vi "3d surface.vi"() -> ()   [LabVIEW 2012]
uses:
  <vilib>/Native 3D Graph/xcontrol/3DPC_SurfacePlot.xctl
  <vilib>/imath/engines/lvmath2/RunTimeEngine/ErrorHandling/NIMS_Finalize Error.vi
  <vilib>/imath/engines/lvmath2/RunTimeEngine/NodeEndStatement/NIMS_NodeEndStatement_Output.vi
  <instcachedir>/0/NIMS_NodeEndStatement_Output_53EC0D466D134D7ABD903AC30B43404B.lvgen/NIMS_NodeEndStatement_Output_53EC0D466D134D7ABD903AC30B43404B_002.vi
  <vilib>/imath/engines/lvmath2/RunTimeEngine/BuiltInFunctions/peakfcn2d/NIMS_peakfcn2d(I32S).vi
  <vilib>/imath/engines/lvmath2/RunTimeEngine/ErrorHandling/NIMS_Error From Error Code.vi
  <vilib>/imath/engines/lvmath2/RunTimeEngine/BuiltInFunctions/surface/NIMS_surface(RM, RM).vi
  <vilib>/imathl/engines/lvmath/Functions/Error Handling/Create Error.vi
panel:
  out "3D Graph":refnum<class "Base Datatype.lvclass">[](xcontrol) caption="三维图形"
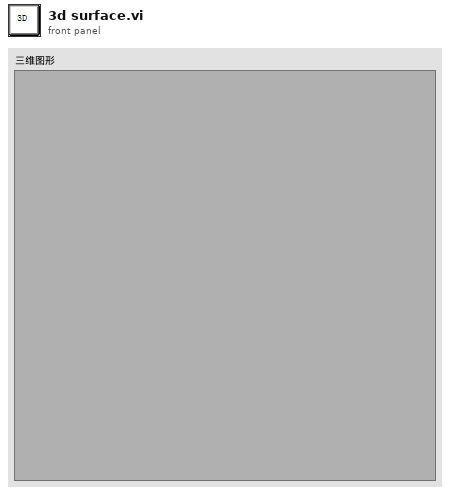
[diagram p1: front panel]
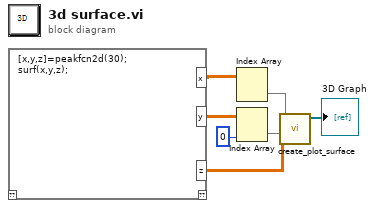
[diagram p0: block diagram]
diagram:
  n1 = mathscript code="[x,y,z]=peakfcn2d(30);\nsurf(x,y,z);"() -> ("x"=w7:dbl[][], "y"=w5:dbl[][], "z"=w3:dbl[][])  [unwired: 1 in, 1 out]
  n2 = Index Array(array=w7) -> (element=w6:dbl[])  [unwired: 2 in]
  n3 = Index Array(array=w5, index (col)=0 ("禁用的索引 (列)")) -> (element=w4:dbl[])  [unwired: 1 in]
  n4 = call <vilib>:"create_plot_surface.vi"("z matrix"=w3, "y vector"=w4, "x vector"=w6) -> ("plots out"=→"3D Graph":refnum<class "Base Datatype.lvclass">[])  [unwired: 2 in, 6 out]
